vi "HIOKI PW3390 Initialize LAN.vi"(0 "IP Address":string="192.168.1.1", 1 "ID Query (T: Yes)":bool=TRUE, 2 "Reset (F: No)":bool, 11 "error in (no error)":errorcluster) -> (4 "VISA Resource out":refnum<visa-resource-name>, 6 "ID":string, 15 "error out":errorcluster)   [LabVIEW 2018]
doc: "Starts the communication with the PW3390 device. This instance can select from the \"HIOKI PW3390 Initialize.vi (Polymorphic VI)\"."
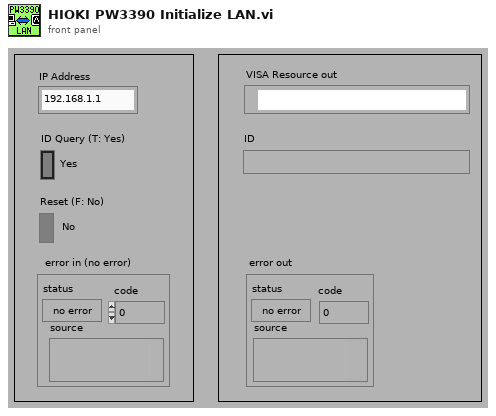
[diagram p1: front panel]
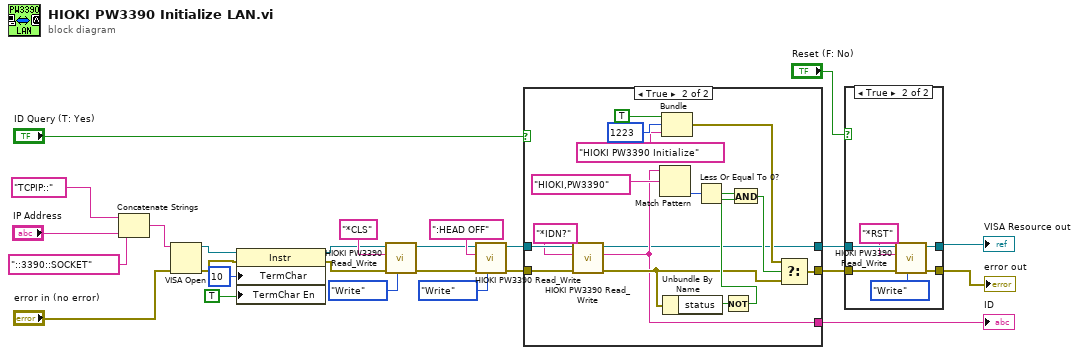
[diagram p0: block diagram]
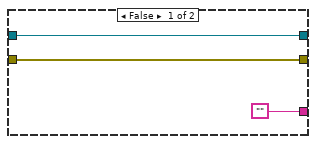
[diagram p3: hidden frame]
diagram:
  n1 = Concatenate Strings("TCPIP::", "IP Address", "::3390::SOCKET") -> (w11:string)
  n2 = VISA Open(error in (no error)="error in (no error)", VISA resource name=w11) -> (VISA resource name=w4:refnum<visa-resource-name>, error out=w3:errorcluster)  [unwired: 3 in]
  n3 = property class="Instr"(reference=w4, error in=w3, "TermChar"=u8 10 ("Message Based Settings:Termination Character"), "TermChar En"=TRUE ("Message Based Settings:Termination Character Enable")) -> (reference out=w2:refnum<visa-resource-name>, error out=w1:errorcluster)
  n4 = call "HIOKI PW3390 Read_Write.vi"("Read/Write"=enum16{"Read", "Write"}."Write", "error in (no error)"=w1, "data in"="*CLS", "VISA Resource"=w2) -> ("error out"=w12:errorcluster, "VISA Resource out"=w13:refnum<visa-resource-name>)  [unwired: 5 in, 1 out]
  n5 = call "HIOKI PW3390 Read_Write.vi"("Read/Write"=enum16{"Read", "Write"}."Write", "error in (no error)"=w12, "data in"=":HEAD OFF", "VISA Resource"=w13) -> ("error out"=w18:errorcluster, "VISA Resource out"=w17:refnum<visa-resource-name>)  [unwired: 5 in, 1 out]
  n6 = case shown="True" "ID Query (T: Yes)" {
    tunnel: w18 -> [w28 w34]
    tunnel: [w28 w42] -> w25
    tunnel: w17 -> [w29 w35]
    tunnel: [w29 w30] -> w26
    tunnel: ["" ("ÇÝÝÊÞ¯Ì§") w31] -> w23
    frame False {
    }
    frame True {
      n7 = call "HIOKI PW3390 Read_Write.vi"("error in (no error)"=w34, "data in"="*IDN?", "VISA Resource"=w35) -> ("error out"=w33:errorcluster, "data out"=w31:string, "VISA Resource out"=w30:refnum<visa-resource-name>)  [unwired: 6 in]
      n8 = Match Pattern(string=w31, regular expression="HIOKI,PW3390") -> (offset past match=w45:i32)  [unwired: 1 in, 3 out]
      n9 = Bundle("status"=TRUE, "code"=1223, "source"="HIOKI PW3390 Initialize") -> (w41:errorcluster)  [unwired: 1 in]
      n10 = Unbundle By Name(w33) -> ("status"=w37:bool)
      n11 = Less Or Equal To 0?(x=w45) -> (x <= 0?=w44:bool)
      n12 = Not(x=w37) -> (.not. x?=w36:bool)
      n13 = And(x=w44, y=w36) -> (x .and. y?=w43:bool)
      n14 = Select(t=w41, s=w43, f=w33) -> (s? t:f=w42:errorcluster)
    }
  }
  "ID" <- w23
  n15 = case shown="True" "Reset (F: No)" {
    tunnel: w26 -> [w47 w54]
    tunnel: w25 -> [w48 w53]
    tunnel: [w48 w52] -> w24
    tunnel: [w47 w49] -> w7
    frame False {
    }
    frame True {
      n16 = call "HIOKI PW3390 Read_Write.vi"("Read/Write"=enum16{"Read", "Write"}."Write", "error in (no error)"=w53, "data in"="*RST", "VISA Resource"=w54) -> ("error out"=w52:errorcluster, "VISA Resource out"=w49:refnum<visa-resource-name>)  [unwired: 5 in, 1 out]
    }
  }
  "error out" <- w24
  "VISA Resource out" <- w7
